vi "Actor Core.vi"(8 "error in":errorcluster, 11 "Nested in":refnum<class "Chat Window Interface.lvclass">) -> (0 "error out":errorcluster, 3 "Actor out":refnum<class "Actor.lvclass">)   [LabVIEW 2015, in "Chat Window Interface.lvlib" / "Chat Window Interface.lvclass"]
doc: "(<B>Filename</B>: Actor Framework.lvlib:Actor.lvclass:Actor Core.vi)\n\nReceives messages to the actor, reacts to them, and initiates any error handling that may shut the actor down.\n\nDescendant classes may override this VI to append parallel tasks for the actor to complete while it handles messages. Overrides use the Call Parent Method node."
uses:
  Chat Window Interface.lvclass
  <vilib>/ActorFramework/Actor/Actor.lvclass
  <vilib>/ActorFramework/Stop Msg/Stop Msg.lvclass
  Chat Window UI Controller/Chat Window UI Controller Messages/Send Status Updated Msg/Send Status Updated Msg.lvclass
  Chat Window UI Controller/Chat Window UI Controller Messages/Send Send Direct Message Msg/Send Send Direct Message Msg.lvclass
  Controls/Message Control.ctl
  Chat Window UI Controller/Chat Window UI Controller/Chat Window UI Controller.lvclass
panel:
  in  "My Status":string
  in  "Message":string
  in  "Send Message":bool
  in  "To":string(combo)
  out "Who's Online":string[](array[string])
  out "Messages":string
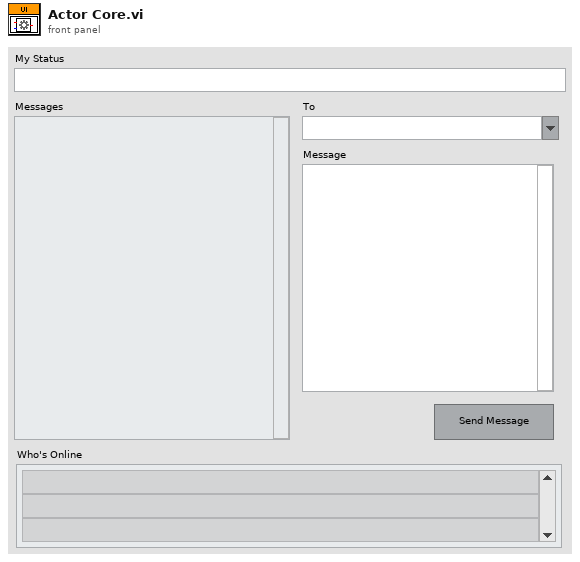
[diagram p1: front panel]
types:
  T1 = cluster{"Stop":refnum<user-event>, "Messages":refnum<user-event>, "OnlineStatus":refnum<user-event>}
  T2 = typedef "Message Control.ctl" = cluster{"From":string, "To":string, "Message":string}
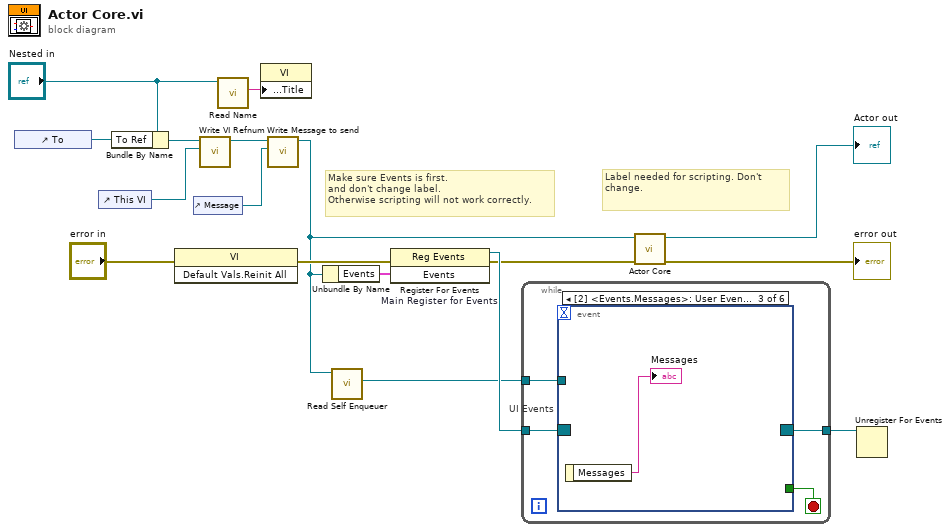
[diagram p0: block diagram]
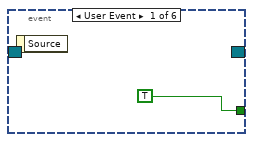
[diagram p2: hidden frame]
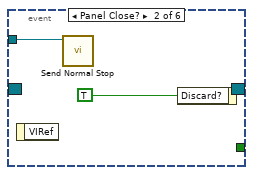
[diagram p3: hidden frame]
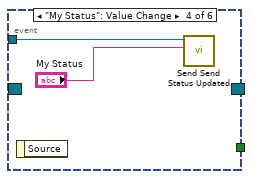
[diagram p4: hidden frame]
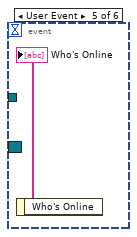
[diagram p5: hidden frame]
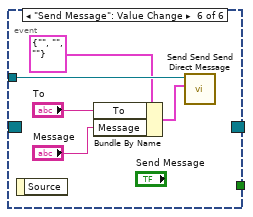
[diagram p6: hidden frame]
diagram:
  # "Label needed for scripting. Don't change."
  # "Make sure Events is first.\nand don't change label.\nOtherwise scripting will not work correctly."
  n1 = control-ref of="To"() -> (w8:refnum<vi>)
  n2 = control-ref of="This VI"() -> (w4:refnum<vi>)
  n3 = Bundle By Name(cluster="Nested in", "To Ref"=w8) -> (w5:refnum<class "Chat Window Interface.lvclass">)
  n4 = invoke class="VI" method="Default Vals.Reinit All"(error in="error in") -> (error out=w9:errorcluster)  [unwired: 2 in, 2 out]
  n5 = control-ref of="Message"() -> (w3:refnum<vi>)
  n6 = call "Write VI Refnum.vi"("VI Refnum"=w4, "Chat Window UI Controller in"=w5) -> ("Chat Window UI Controller out"=w2:refnum<class "Chat Window Interface.lvclass">)  [unwired: 8 in, 1 out]
  n7 = call "Read Name.vi"("Chat Window UI Controller in"="Nested in") -> ("Name"=w6:string)  [unwired: 8 in, 2 out]
  n8 = property class="VI"("Front Panel.Title"=w6) -> ()  [unwired: 2 in, 2 out]
  n9 = call "Write Message to send.vi"("Message to send"=w3, "Chat Window UI Controller in"=w2) -> ("Chat Window UI Controller out"=w1:refnum<class "Chat Window Interface.lvclass">)  [unwired: 8 in, 1 out]
  n10 = Unbundle By Name(w1) -> ("Events"=w14:T1)
  n11 = call <vilib>:"Read Self Enqueuer.vi"("Actor"=w1) -> ("Self Enqueuer"=w12:refnum<class "Message Enqueuer.lvclass">)  [unwired: 10 in]
  n12 = register-events "Main Register for Events"(error in=w9, w14) -> (reference out=w15:refnum<event-registration>, error out=w11:errorcluster)  [unwired: 1 in]
  n13 = while {
    tunnel: w15 -> [w21]
    tunnel: [w19] -> w13
    tunnel: w12 -> [w18]
    stop <- w20 stop-if-true
    n14 = event "UI Events" shown="[2] <Events.Messages>: User Event" {
      selector: w21 -> [_ _ _ _ _ _]
      dyn-events: [_ _ _ _ _ _] -> w19
      timeout: _ -> [_ _ _ _ _ _]
      tunnel: [TRUE _ _ _ _ _] -> w20
      tunnel: w18 -> [_ w23 _ w27 _ w33]
      event User Event {
        n15 = event-data() -> ()  [unwired: 1 in, 1 out]
      }
      event Panel Close? {
        n16 = event-data() -> ()  [unwired: 1 in, 1 out]
        n17 = call <vilib>:"Send Normal Stop.vi"("Message Enqueuer"=w23) -> ()  [unwired: 10 in, 1 out]
        n18 = event-data("Discard?"=TRUE) -> ()  [unwired: 1 in, 1 out]
      }
      event User Event {
        n19 = event-data() -> ("Messages"=→"Messages":string)  [unwired: 1 in]
      }
      event "My Status": Value Change {
        n20 = event-data() -> ()  [unwired: 1 in, 1 out]
        n21 = call "Send Send Status Updated.vi"("Status"="My Status", "Message Enqueuer"=w27) -> ()  [unwired: 8 in, 2 out]
      }
      event User Event {
        n22 = event-data() -> ("Who's Online"=→"Who's Online":string[])  [unwired: 1 in]
      }
      event "Send Message": Value Change {
        n23 = event-data() -> ()  [unwired: 1 in, 1 out]
        n24 = Bundle By Name(cluster=T2 {"From"="", "To"="", "Message"=""} ("Message"), "To"="To", "Message"="Message") -> (w31:T2)
        n25 = call "Send Send Send Direct Message.vi"("Message"=w31, "Message Enqueuer"=w33) -> ()  [unwired: 8 in, 2 out]
      }
    }
  }
  n26 = call-parent "Actor Core.vi"("error in"=w11, "Actor in"=w1) -> ("error out"=→"error out":errorcluster, "Actor out"=→"Actor out":refnum<class "Actor.lvclass">)  [unwired: 8 in]
  n27 = Unregister For Events(event registration refnum=w13) -> ()  [unwired: 1 in, 1 out]
